vi "InitializeCNet.vi"(2 "NIN":u32, 3 "error in (no error)":errorcluster) -> (0 "ptr":i64, 1 "error out":errorcluster)   [LabVIEW 2016, in "CNet.lvlib"]
uses:
  CNet.lvlib
  Users/jg754/Documents/Visual Studio 2015/Projects/CLearn/x64/Release/CLearn.dll
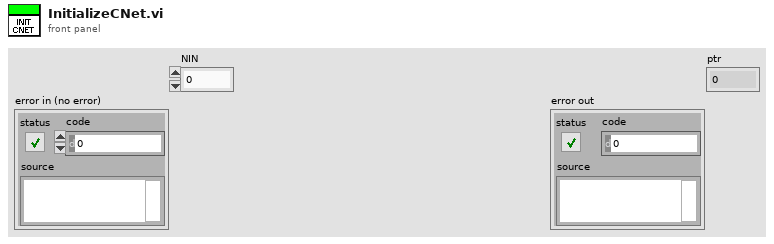
[diagram p1: front panel]
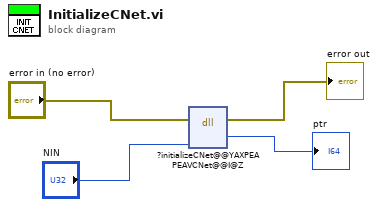
[diagram p0: block diagram]
diagram:
  n1 = dll-call lib="C:/Users/jg754/Documents/Visual Studio 2015/Projects/CLearn/x64/Release/CLearn.dll" fn="?initializeCNet@@YAXPEAPEAVCNet@@I@Z"(error in="error in (no error)", "NIN"="NIN") -> (error out=→"error out":errorcluster, "ptr"=→"ptr":i64)  [unwired: 5 in, 1 out]
